vi "Configure Display.vi"(0 "VISA resource name":refnum<visa-resource-name>, 1 "Display Brightness (2: 75%)":u16(ring)=2 items=["25%", "50%", "75%", "100%"], 5 "Field (1)":dbl=1.0 min=1.0 max=4.0 step=1.0, 7 "Item to Display (0: None)":u16(ring) items=["None", "Input A", "Input B", "Setpoint", "Heater Output"], 9 "Source (0: Kelvin)":u16(ring) items=["Kelvin", "Celsius", "Sensor Units", "Linear Data", "Min Data", "Max Data"], 11 "error in (no error)":errorcluster) -> (4 "VISA resource name out":refnum<visa-resource-name>, 15 "error out":errorcluster)   [LabVIEW 2013, in "Lake Shore Cryotronics 331.lvlib"]
doc: "This VI Configures the parameters of the front panel display."
uses:
  Lake Shore Cryotronics 331.lvlib
panel:
  # "Displayed Field Parameters"
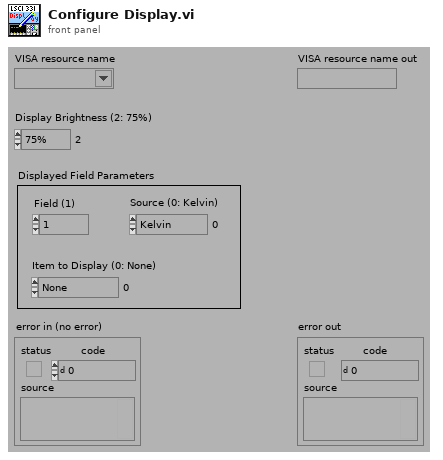
[diagram p1: front panel]
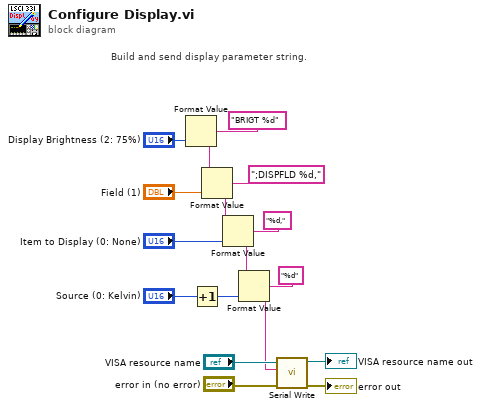
[diagram p0: block diagram]
diagram:
  # "Build and send display parameter string."
  n1 = Format Value(format string="BRIGT %d", value (0)="Display Brightness (2: 75%)") -> (output string=w5:string)  [unwired: 1 in]
  n2 = Increment(x="Source (0: Kelvin)") -> (x+1=w16:u16)
  n3 = Format Value(string ("")=w5, format string=";DISPFLD %d,", value (0)="Field (1)") -> (output string=w4:string)
  n4 = Format Value(string ("")=w4, format string="%d,", value (0)="Item to Display (0: None)") -> (output string=w2:string)
  n5 = Format Value(string ("")=w2, format string="%d", value (0)=w16) -> (output string=w1:string)
  n6 = call "Serial Write.vi"("error in (no error)"="error in (no error)", "Write Buffer (\"\")"=w1, "VISA resource name"="VISA resource name") -> ("error out"=→"error out":errorcluster, "VISA resource name out"=→"VISA resource name out":refnum<visa-resource-name>)  [unwired: 6 in, 1 out]
